vi "RLC READ DINAMICO.vi"(7 "Boolean":bool) -> (0 "MEASURE R [Ohm ]":dbl, 3 "MEASURE C [F ]":dbl)   [LabVIEW 2011]
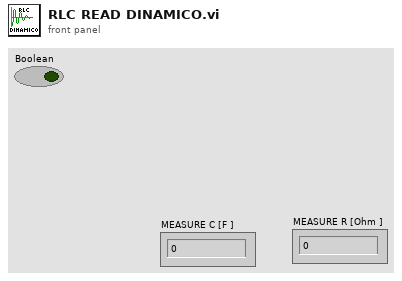
[diagram p1: front panel]
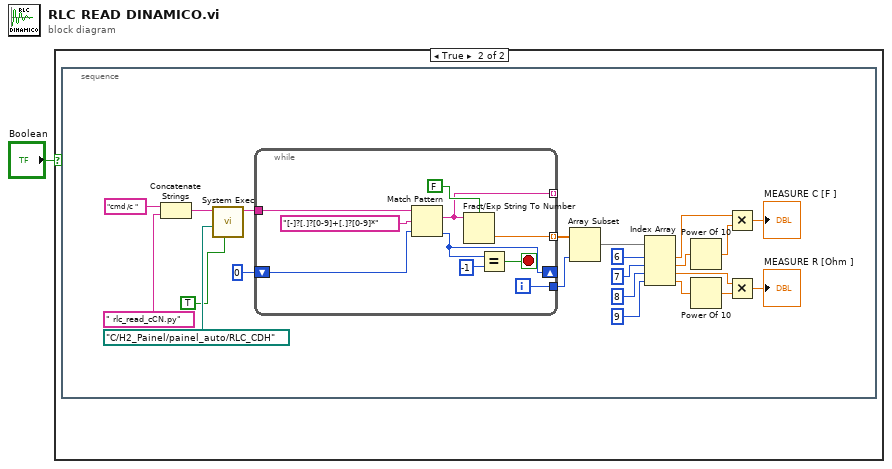
[diagram p0: block diagram]
diagram:
  n1 = case shown="True" "Boolean" {
    frame False {
    }
    frame True {
      n2 = stacked-sequence {
        frame #0 {
          n3 = Concatenate Strings("cmd /c ", " rlc_read_cCN.py" ("String")) -> (w4:string)
          n4 = call <vilib>:"System Exec.vi"("run minimized? (F)"=TRUE, "working directory"=path "C:/H2_Painel/painel_auto/RLC_CDH" ("Path"), "command line"=w4) -> ("standard output"=w12:string)  [unwired: 5 in, 3 out]
          n5 = while {
            tunnel: [w33] -> w19
            shift-left: 0 -> [w28]
            shift-right: [w27] -> _
            tunnel: [w31] -> w18 mode=indexing
            tunnel: [w25] -> _ mode=indexing
            tunnel: w12 -> [w24]
            i -> [w33]
            stop <- w30 stop-if-true
            n6 = Match Pattern(string=w24, regular expression="[-]?[.]?[0-9]+[.]?[0-9]*", offset (0)=w28) -> (match substring=w25:string, offset past match=w27:i32)  [unwired: 2 out]
            n7 = Fract/Exp String To Number(use system decimal point (T)=FALSE, string=w25) -> (number=w31:dbl)  [unwired: 2 in, 1 out]
            n8 = Equal?(x=w27, y=-1) -> (x = y?=w30:bool)
          }
          n9 = Array Subset(array=w18, length=w19) -> (w20:dbl[])  [unwired: 1 in]
          n10 = Index Array(array=w20, index #1=6, index #2=7, index #3=8 ("index"), index #4=9 ("index")) -> (element #1=w13:dbl, element #2=w14:dbl, element #3=w8:dbl, element #4=w7:dbl)
          n11 = Power Of 10(x=w14) -> (10^x=w21:dbl)
          n12 = Power Of 10(x=w7) -> (10^x=w9:dbl)
          n13 = Multiply(x=w13, y=w21) -> (x*y=→"MEASURE C [F ]":dbl)
          n14 = Multiply(x=w8, y=w9) -> (x*y=→"MEASURE R [Ohm ]":dbl)
        }
      }
    }
  }
